vi "search_database.vi"() -> ()   [LabVIEW 2023]
uses:
  user_details.ctl
  search_option.ctl
panel:
  in  "stop":bool
  out "Search Time (ms)":dbl format="%.3f"
  in  "Search Option":T1
  in  "Valid Upto":dbl
  in  "Card Number":string
  in  "Card Holder Name":string
  out "Card Number Search Result":T2
  out "Valid Upto Search Result":T2[](array[typedef])
  out "Card Holder Name Search Result":T2[](array[typedef])
  in  "Account Details":T2[](array[typedef])=[{"Card Number"="11", "Card Holder Name"="Tom", "Valid Upto"=2026.0}, {"Card Number"="12", "Card Holder Name"="Com", "Valid Upto"=2026.0}, {"Card Number"="13", "Card Holder Name"="John", "Valid Upto"=2039.0}, {"Card Number"="14", "Card Holder Name"="Joe", "Valid Upto"=2050.0}, {"Card Number"="15", "Card Holder Name"="Burton", "Valid Upto"=2029.0}, {"Card Number"="16", "Card Holder Name"="low", "Valid Upto"=2060.0}]
  # "DATABASE"
  # "SEARCH BOX"
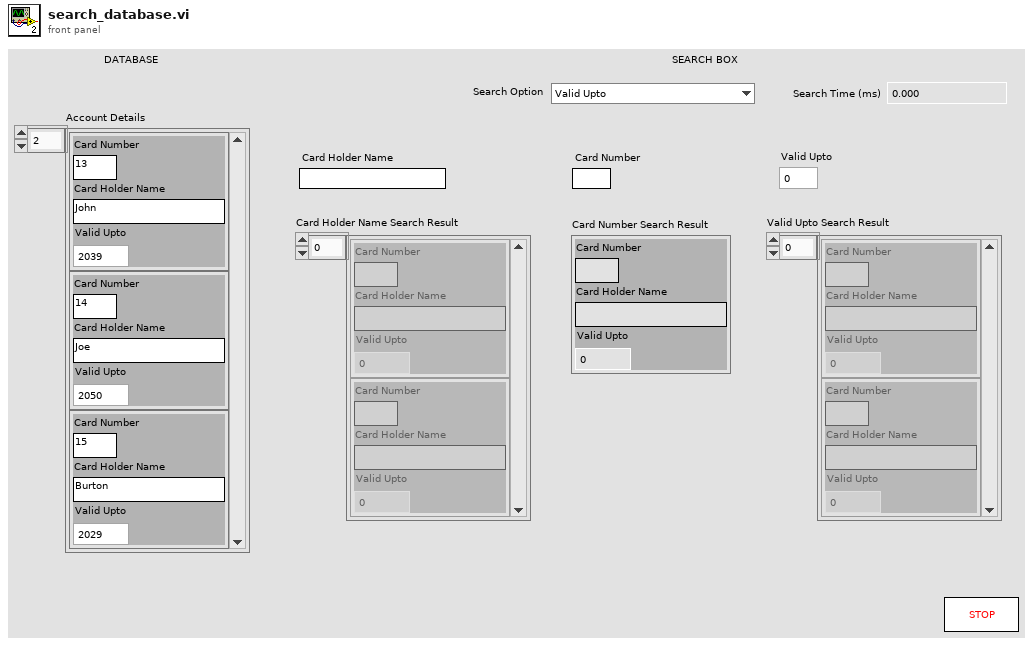
[diagram p1: front panel]
types:
  T1 = typedef "search_option.ctl" = enum16{"Valid Upto", "Card Number", "Card Holder Name"}
  T2 = typedef "user_details.ctl" = cluster{"Card Number":string, "Card Holder Name":string, "Valid Upto":dbl}
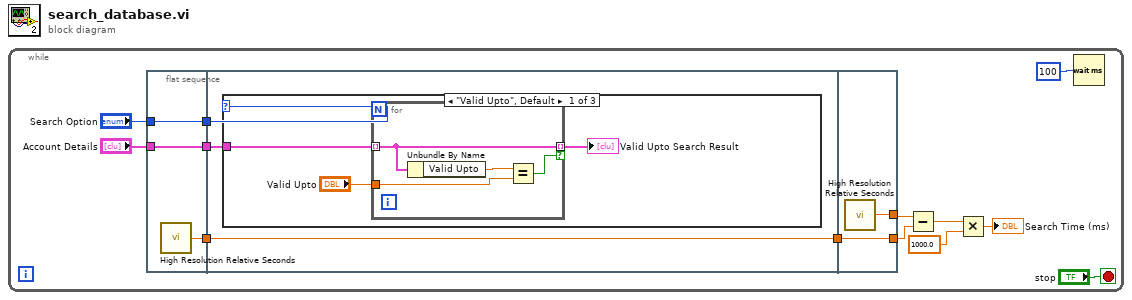
[diagram p0: block diagram]
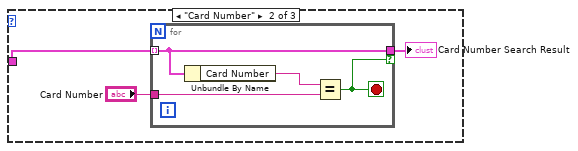
[diagram p2: hidden frame]
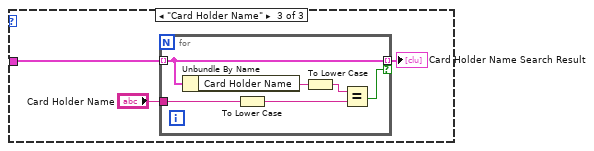
[diagram p3: hidden frame]
diagram:
  n1 = while {
    stop <- "stop" stop-if-true
    n2 = flat-sequence {
      tunnel: "Account Details" -> [w15]
      tunnel: "Search Option" -> [w16]
      tunnel: [w16] -> w9
      tunnel: [w15] -> w8
      tunnel: [w14] -> w2
      tunnel: w9 -> [w19]
      tunnel: w8 -> [w18]
      tunnel: [w17] -> w3
      tunnel: w2 -> [w17]
      tunnel: [w44] -> w7
      tunnel: [w43] -> w1
      tunnel: w3 -> [w43]
      frame #0 {
        n3 = call <vilib>:"High Resolution Relative Seconds.vi"() -> ("relative seconds"=w14:dbl)
      }
      frame #1 {
        n4 = case shown="\"Valid Upto\", Default" w19 {
          tunnel: w18 -> [w22 w29 w36]
          frame "Valid Upto", Default {
            n5 = for {
              tunnel: w22 -> [w23] mode=indexing
              tunnel: "Valid Upto" -> [w25]
              tunnel: [w23] -> w20 mode=indexing if=w26
              n6 = Unbundle By Name(w23) -> ("Valid Upto"=w24:dbl)
              n7 = Equal?(x=w24, y=w25) -> (x = y?=w26:bool)
            }
            "Valid Upto Search Result" <- w20
          }
          frame "Card Number" {
            n8 = for {
              tunnel: w29 -> [w31] mode=indexing
              tunnel: "Card Number" -> [w33]
              tunnel: [w31] -> w27 if=w30
              stop <- w30 stop-if-true
              n9 = Unbundle By Name(w31) -> ("Card Number"=w32:string)
              n10 = Equal?(x=w32, y=w33) -> (x = y?=w30:bool)
            }
            "Card Number Search Result" <- w27
          }
          frame "Card Holder Name" {
            n11 = for {
              tunnel: w36 -> [w39] mode=indexing
              tunnel: "Card Holder Name" -> [w41]
              tunnel: [w39] -> w34 mode=indexing if=w42
              n12 = Unbundle By Name(w39) -> ("Card Holder Name"=w40:string)
              n13 = To Lower Case(string=w41) -> (all lower case string=w38:string)
              n14 = To Lower Case(string=w40) -> (all lower case string=w37:string)
              n15 = Equal?(x=w37, y=w38) -> (x = y?=w42:bool)
            }
            "Card Holder Name Search Result" <- w34
          }
        }
      }
      frame #2 {
        n16 = call <vilib>:"High Resolution Relative Seconds.vi"() -> ("relative seconds"=w44:dbl)
      }
    }
    n17 = Subtract(x=w7, y=w1) -> (x-y=w6:dbl)
    n18 = Multiply(x=w6, y=1000.0) -> (x*y=→"Search Time (ms)":dbl)
    n19 = Wait (ms)(milliseconds to wait=u32 100) -> ()  [unwired: 1 out]
  }
